vi "MAX31855 Thermocouple Sensor.vi"   [LabVIEW 2014]
uses:
  QwaveSys_Interface/QwaveSys_Interface.lvlib
  QwaveSys_ESP8266/QwaveSys_ESP8266.lvlib
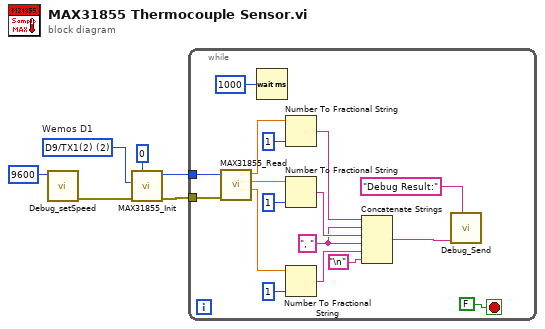
[diagram p0: block diagram]
diagram:
  w1 = u8 2 items=["D0-RX(3)"=3, "D1-TX(1)"=1, "D2(16)"=16, "D3/D15/SCL(5)"=5, "D4/D14/SDA(4)"=4, "D5/D13/SCK(14)-(LED)"=14, "D6/D12/MISO(12)"=12, "D7/D11/MOSI(13)"=13, "D8(0)"=0, "D9/TX1(2)"=2, "D10/SS (15)"=15, "ADC0,(17)"=17]  # Wemos D1
  n1 = call "Debug_setSpeed.vi"("Speed"=u32 9600) -> ("error out"=w4:errorcluster)  [unwired: 10 in]
  n2 = call "MAX31855_Init.vi"("error in"=w4, "CS"=w1, "Interface (0-4)"=u8 0) -> ("error out"=w6:errorcluster, "Instance"=w5:u8)  [unwired: 7 in]
  n3 = while {
    tunnel: w6 -> [w23]
    tunnel: w5 -> [w9]
    stop <- FALSE stop-if-true
    w11 = ", " ("string")
    n4 = call "MAX31855_Read.vi"("Instance"=w9, "error in (no error)"=w23) -> ("Farenheit"=w13:dbl, "Celsius"=w20:dbl, "Internal Temp"=w21:dbl)  [unwired: 6 in, 1 out]
    n5 = Wait (ms)(milliseconds to wait=u32 1000) -> ()  [unwired: 1 out]
    n6 = Number To Fractional String(number=w21, precision (6)=i16 1) -> (F-format string=w19:string)  [unwired: 2 in]
    n7 = Number To Fractional String(number=w20, precision (6)=i16 1) -> (F-format string=w18:string)  [unwired: 2 in]
    n8 = Number To Fractional String(number=w13, precision (6)=i16 1) -> (F-format string=w10:string)  [unwired: 2 in]
    n9 = Concatenate Strings(w19, w11, w18, w11, w10, "\n" ("Line Feed Constant")) -> (w8:string)
    n10 = call "Debug_Send.vi"("Name"="Debug Result:", "DATA"=w8) -> ()  [unwired: 10 in]
  }
